vi "Shutdown.vi"(8 "error in (no error)":errorcluster, 11 "DAQ_QPT_Throlab in":refnum<class "DAQ_QPT_Throlab.lvclass">) -> (0 "error out":errorcluster, 3 "DAQ_QPT_Throlab out":refnum<class "DAQ_QPT_Throlab.lvclass">)   [LabVIEW 2020, in "DAQ_QPT_Throlab.lvlib" / "DAQ_QPT_Throlab.lvclass"]
uses:
  DAQ_QPT_Throlab.lvclass
  DAQ_QPT_Throlab.lvclass/DAQ_QPT_Throlab.ctl
  Hardware Abstraction Layer/Component/DAQ/DAQ/DAQ.lvclass
  Dependency/TIRF-Lock.dll
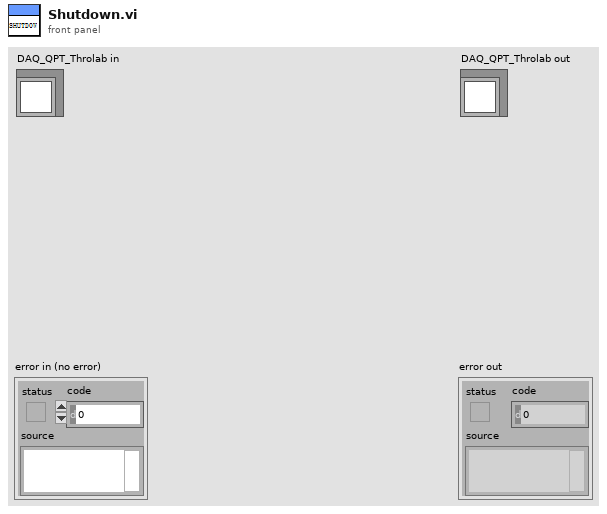
[diagram p1: front panel]
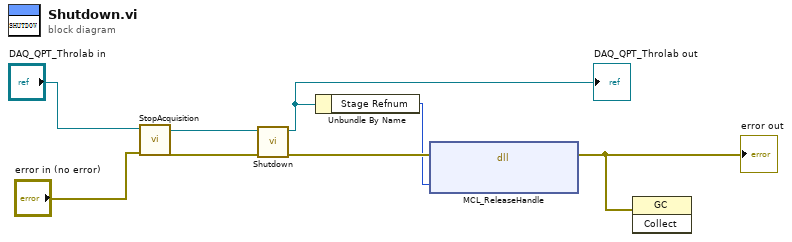
[diagram p0: block diagram]
diagram:
  n1 = call-dynamic "StopAcquisition.vi"("error in (no error)"="error in (no error)", "Device in"="DAQ_QPT_Throlab in") -> ("error out"=w7:errorcluster, "Device out"=w5:refnum<class "DAQ_QPT_Throlab.lvclass">)  [unwired: 8 in]
  n2 = call-parent "Shutdown.vi"("error in (no error)"=w7, "Device in"=w5) -> ("error out"=w4:errorcluster, "Device out"=w3:refnum<class "DAQ_QPT_Throlab.lvclass">)  [unwired: 8 in]
  "DAQ_QPT_Throlab out" <- w3
  n3 = Unbundle By Name(w3) -> ("Stage Refnum"=w2:i32)
  n4 = dll-call lib="E:/Development/DevHardSoftware/MicroscopyFramework/Model/Hardware Layer/Real Hardware/DAQ_QPT_Throlab/DAQ_QPT_Throlab/Dependency/TIRF-Lock.dll" fn="MCL_ReleaseHandle"(error in=w4, "handle"=w2) -> (error out=w1:errorcluster)  [unwired: 3 in, 2 out]
  "error out" <- w1
  n5 = invoke class="GC" method="Collect"(error in=w1) -> ()  [unwired: 2 in, 3 out]
